vi "poly_cast_variant_array_I8.vi"(2 "variant":variant) -> (7 "data (empty)":i8[](array[numeric]))   [LabVIEW 2015]
doc: "This vi attempts to cast a variant to data. The data is set to default value if an error occurs. This vi is intended to be used as a convenience tool when the data type is unambigous.\n\nWritten by Marcin Konowalczyk\nTimmel Group @ Oxford University"
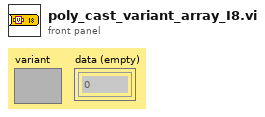
[diagram p1: front panel]
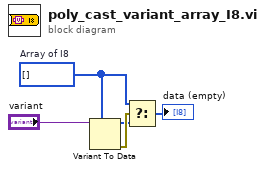
[diagram p0: block diagram]
diagram:
  w1 = i8[] []  # Array of I8
  n1 = Variant To Data(type=w1, Variant="variant") -> (data=w3:i8[], error out=w4:errorcluster)  [unwired: 1 in]
  n2 = Select(t=w1, s=w4, f=w3) -> (s? t:f=→"data (empty)":i8[])
